vi "1_04.vi"() -> ()   [LabVIEW 2018]
panel:
  out "Waveform Chart":dbl[](graph)
  in  "Amplitud":dbl=5.0
  in  "Frecuencia":dbl=1000.0
  in  "Muestras":dbl=2.0
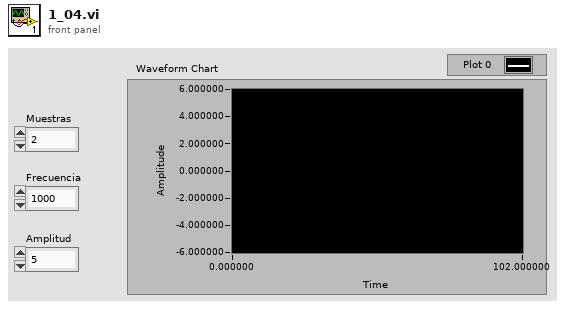
[diagram p1: front panel]
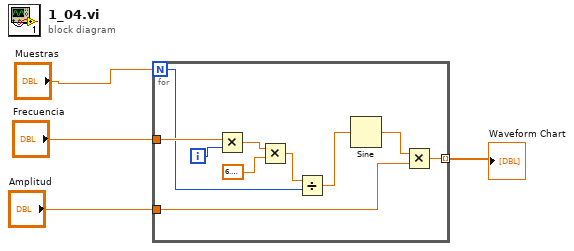
[diagram p0: block diagram]
diagram:
  n1 = for {
    N: "Muestras" -> [w5]
    tunnel: "Frecuencia" -> [w13]
    tunnel: "Amplitud" -> [w8]
    tunnel: [w6] -> w2 mode=indexing
    i -> [w14]
    n2 = Multiply(x=w13, y=w14) -> (x*y=w11:dbl)
    n3 = Multiply(x=w11, y=6.283185307179586) -> (x*y=w10:dbl)
    n4 = Divide(x=w10, y=w5) -> (x/y=w9:dbl)
    n5 = Sine(x=w9) -> (sin(x)=w7:dbl)
    n6 = Multiply(x=w7, y=w8) -> (x*y=w6:dbl)
  }
  "Waveform Chart" <- w2
